vi "Get User VI Owners.vi"(8 "error in":errorcluster, 11 "User VI Ref":refnum<vi>) -> (0 "error out":errorcluster, 1 "Owner Filename (inc file extension)":string, 2 "Owner Path":path, 3 "User VI Owner Status":T2, 4 "Owner Filename (excluding file extension)":string, 5 "Owner Reference":refnum<vi>, 6 "Virtual Folder Search Output":T1)   [LabVIEW 2022 SP3]
doc: "Gets details about the \"owners\" of the User VI. A VI could be owned by a library (.lvlib), a class (.lvclass) or a project (.lvproj)."
uses:
  Owner Status (enum).ctl
  DFS Output (cluster).ctl
panel:
  # "Development\ncontrols/indicators useful for development and testing, but which are not outputs of the VI"
  # "Input\nInputs to the VI"
  # "Output\nOutputs of the VI"
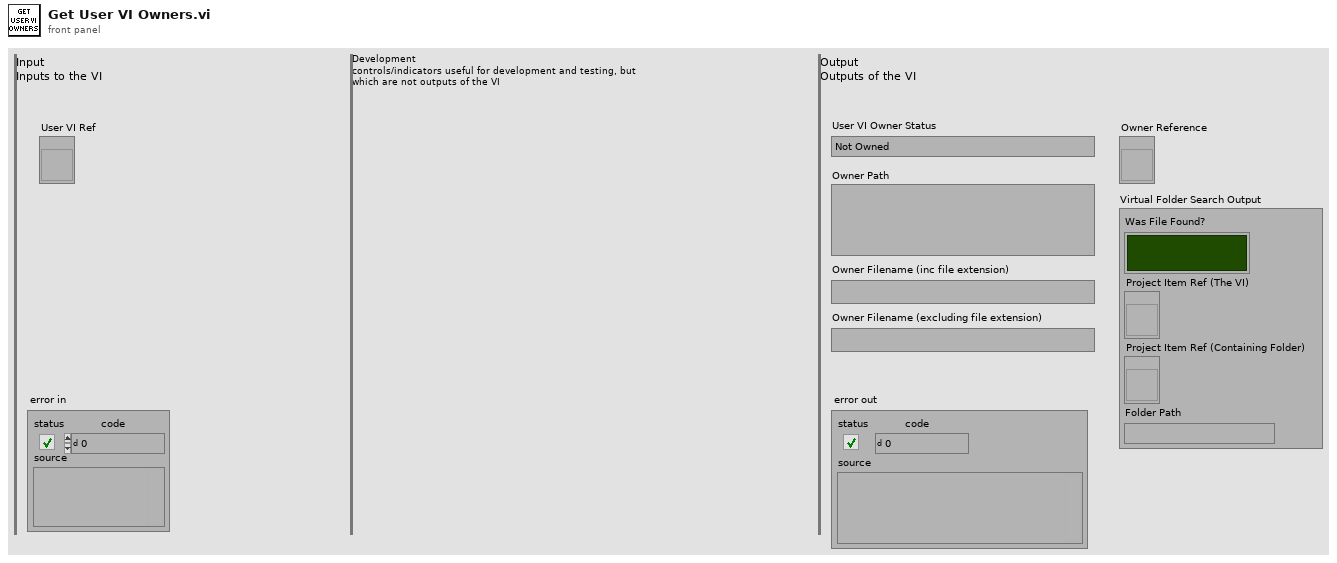
[diagram p1: front panel]
types:
  T1 = typedef "DFS Output (cluster).ctl" = cluster{"Was File Found?":bool, "Project Item Ref (The VI)":refnum<vi>, "Project Item Ref (Containing Folder)":refnum<vi>, "Folder Path":string}
  T2 = typedef "Owner Status (enum).ctl" = enum16{"Not Owned", "Owned by Library (lvlib)", "Owned by Class (lvclass)"}
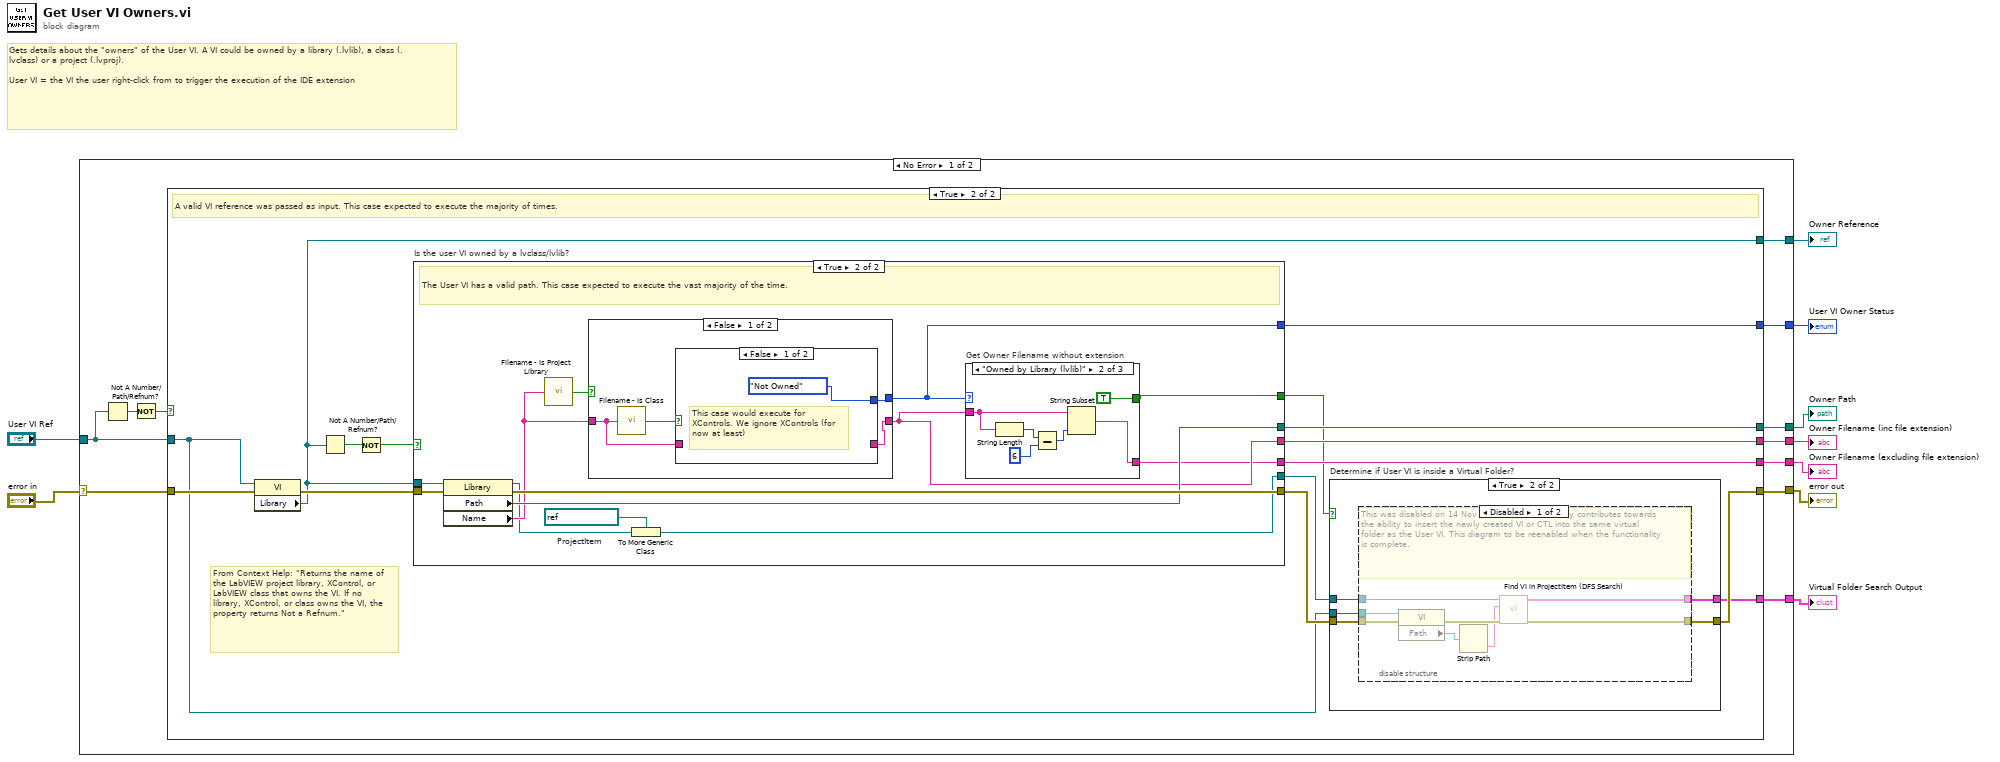
[diagram p0: block diagram]
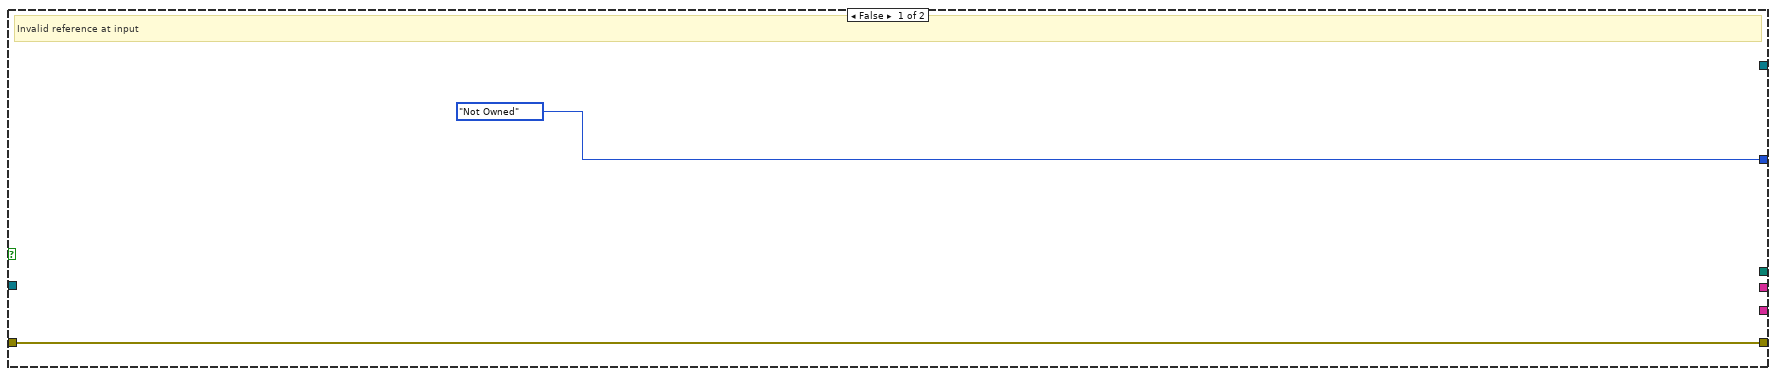
[diagram p2: hidden frame]
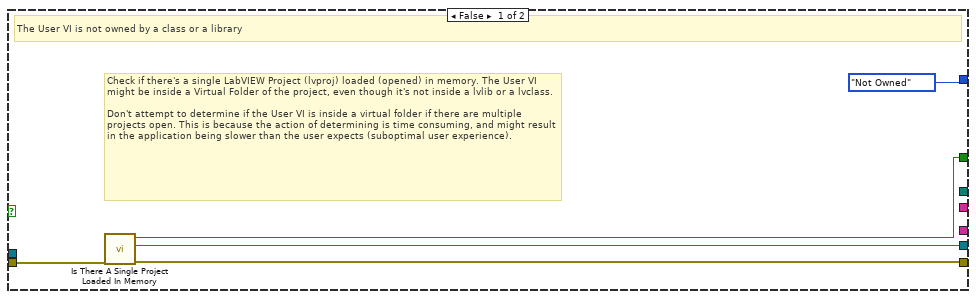
[diagram p5: hidden frame]
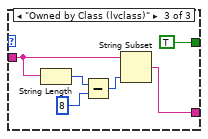
[diagram p7: hidden frame]
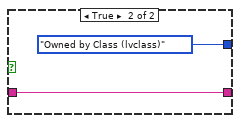
[diagram p8: hidden frame]
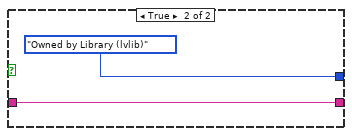
[diagram p9: hidden frame]
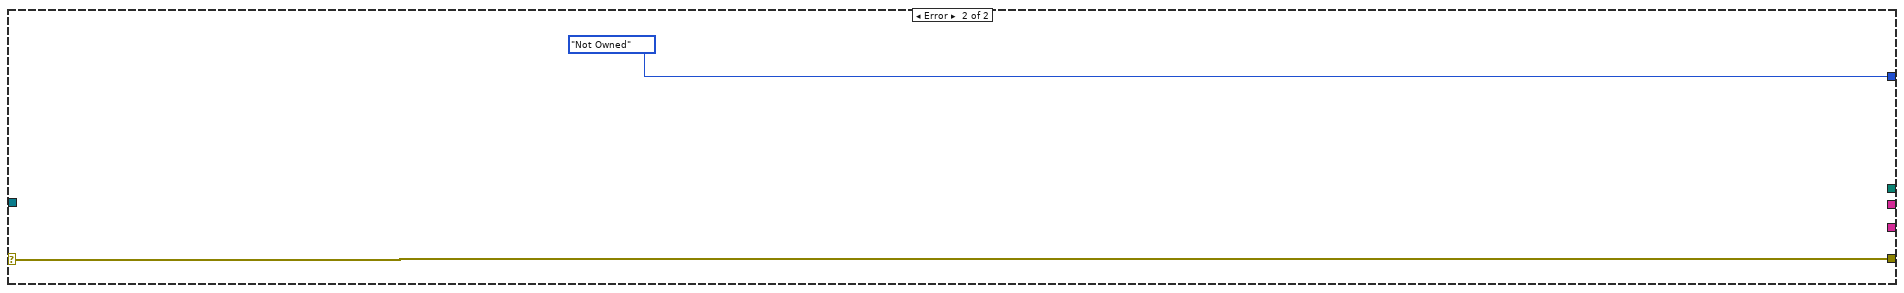
[diagram p10: hidden frame]
diagram:
  # "Gets details about the \"owners\" of the User VI. A VI could be owned by a library (.lvlib), a class (.lvclass) or a project (.lvproj).\n\nUser VI = the VI the user right-click from to trigger the execution of the IDE extension"
  n1 = case shown="No Error" "error in" {
    selector: "error in" -> [w20 w93]
    tunnel: [w19 w93] -> w8
    tunnel: "User VI Ref" -> [w18 _]
    tunnel: [w15 Owner_Status_(enum)."Not Owned" ("Owner Status")] -> w6
    tunnel: [w14 _] -> w5
    tunnel: [w13 _] -> w4
    tunnel: [w12 _] -> w3
    tunnel: [w11 _] -> w2
    tunnel: [w10 _] -> w1
    frame No Error {
      n2 = Not A Number/Path/Refnum?(number/path/refnum=w18) -> (NaN/Path/Refnum?=w17:bool)
      n3 = Not(x=w17) -> (.not. x?=w16:bool)
      n4 = case shown="True" w16 {
        tunnel: w20 -> [w22 w37]
        tunnel: [w22 w27] -> w19
        tunnel: w18 -> [_ w24]
        tunnel: [Owner_Status_(enum)."Not Owned" ("Owner Status") w34] -> w15
        tunnel: [_ w32] -> w14
        tunnel: [_ w31] -> w13
        tunnel: [_ w30] -> w12
        tunnel: [_ w29] -> w11
        tunnel: [_ w23] -> w10
        frame False {
          # "Invalid reference at input"
        }
        frame True {
          # "From Context Help: \"Returns the name of the LabVIEW project library, XControl, or LabVIEW class that owns the VI. If no library, XControl, or class owns the VI, the property returns Not a Refnum.\""
          # "A valid VI reference was passed as input. This case expected to execute the majority of times."
          n5 = property class="VI"(reference=w24, error in=w37) -> (error out=w33:errorcluster, "Library"=w29:refnum<vi>)  [unwired: 1 out]
          n6 = Not A Number/Path/Refnum?(number/path/refnum=w29) -> (NaN/Path/Refnum?=w36:bool)
          n7 = Not(x=w36) -> (.not. x?=w35:bool)
          n8 = case "Is the user VI owned by a lvclass/lvlib?" shown="True" w35 {
            tunnel: w29 -> [_ w69]
            tunnel: [Owner_Status_(enum)."Not Owned" ("Owner Status") w62] -> w34
            tunnel: w33 -> [w55 w70]
            tunnel: [w56 w68] -> w28
            tunnel: [_ w67] -> w32
            tunnel: [_ w64] -> w31
            tunnel: [_ w63] -> w30
            tunnel: [w54 w61] -> w26
            tunnel: [w53 w58] -> w25
            frame False {
              # "Check if there's a single LabVIEW Project (lvproj) loaded (opened) in memory. The User VI might be inside a Virtual Folder of the project, even though it's not inside a lvlib or a lvclass.\n\nDon't attempt to determine if the User VI is inside a virtual folder if there are multiple projects open. This is because the action of determining is time consuming, and might result in the application being slower than the user expects (suboptimal user experience)."
              # "The User VI is not owned by a class or a library"
              n9 = call "Is There A Single Project Loaded In Memory.vi"("Error In"=w55) -> ("Error Out"=w56:errorcluster, "My Computer ProjectItem Ref"=w53:refnum<vi>, "A Single Project Loaded In Memory?"=w54:bool)  [unwired: 8 in]
            }
            frame True {
              w59 = refnum<vi> refnum  # ProjectItem
              # "The User VI has a valid path. This case expected to execute the vast majority of the time."
              n10 = property class="Library"(reference=w69, error in=w70) -> (reference out=w60:refnum<vi>, error out=w68:errorcluster, "Path"=w67:path, "Name"=w65:string)
              n11 = call "Filename - Is Project Library.vi"("Filename (including file extension)"=w65) -> ("Is Project Library?"=w66:bool)
              n12 = case shown="False" w66 {
                tunnel: [w85 Owner_Status_(enum)."Owned by Library (lvlib)" ("Owner Status")] -> w62
                tunnel: w65 -> [w83 w90]
                tunnel: [w84 w90] -> w64
                frame False {
                  n13 = call "Filename - Is Class.vi"("Filename (including file extension)"=w83) -> ("Is Class?"=w86:bool)
                  n14 = case shown="False" w86 {
                    tunnel: [Owner_Status_(enum)."Not Owned" ("Owner Status") Owner_Status_(enum)."Owned by Class (lvclass)" ("Owner Status")] -> w85
                    tunnel: [_ w88] -> w84
                    tunnel: w83 -> [_ w88]
                    frame False {
                      # "This case would execute for XControls. We ignore XControls (for now at least)"
                    }
                    frame True {
                    }
                  }
                }
                frame True {
                }
              }
              n15 = To More Generic Class(target class=w59, reference=w60) -> (generic class reference=w58:refnum<vi>)
              n16 = case "Get Owner Filename without extension" shown="\"Owned by Library (lvlib)\"" w62 {
                tunnel: w64 -> [_ w76 w82]
                tunnel: [_ w72 w78] -> w63
                tunnel: [_ TRUE TRUE] -> w61
                frame "Not Owned" {
                }
                frame "Owned by Library (lvlib)" {
                  n17 = String Length(string=w76) -> (length=w74:i32)
                  n18 = Subtract(x=w74, y=6) -> (x-y=w75:i32)
                  n19 = String Subset(string=w76, length (rest)=w75) -> (substring=w72:string)  [unwired: 1 in]
                }
                frame "Owned by Class (lvclass)" {
                  n20 = String Length(string=w82) -> (length=w80:i32)
                  n21 = Subtract(x=w80, y=8) -> (x-y=w81:i32)
                  n22 = String Subset(string=w82, length (rest)=w81) -> (substring=w78:string)  [unwired: 1 in]
                }
              }
            }
          }
          n23 = case "Determine if User VI is inside a Virtual Folder?" shown="True" w26 {
            tunnel: w28 -> [w38 w43]
            tunnel: [w38 w42] -> w27
            tunnel: w25 -> [_ w41]
            tunnel: w24 -> [_ w40]
            tunnel: [_ w39] -> w23
            frame False {
            }
            frame True {
              n24 = disable-structure shown="Disabled" {
                disable-tunnel: w43 -> [w51 w52]
                disable-tunnel: [w50 w52] -> w42
                disable-tunnel: w41 -> [w49 _]
                disable-tunnel: w40 -> [w47 _]
                disable-tunnel: [w46 _] -> w39
                frame Disabled {
                  # "This was disabled on 14 Nov 2022. This functionality contributes towards the ability to insert the newly created VI or CTL into the same virtual folder as the User VI. This diagram to be reenabled when the functionality is complete."
                  n25 = property class="VI"(reference=w47, error in=w51) -> (error out=w48:errorcluster, "Path"=w45:path)  [unwired: 1 out]
                  n26 = Strip Path(path=w45) -> (name=w44:string)  [unwired: 1 out]
                  n27 = call "Find VI in ProjectItem (DFS Search).vi"("Error In"=w48, "VI Filename (including extension)"=w44, "Project Item Ref"=w49) -> ("Error Out"=w50:errorcluster, "Search Output"=w46:T1)  [unwired: 7 in]
                }
                frame Enabled {
                }
              }
            }
          }
        }
      }
    }
    frame Error {
    }
  }
  "error out" <- w8
  "User VI Owner Status" <- w6
  "Owner Filename (inc file extension)" <- w4
  "Owner Path" <- w5
  "Owner Filename (excluding file extension)" <- w3
  "Owner Reference" <- w2
  "Virtual Folder Search Output" <- w1
